vi "enum01.vi"() -> ()   [LabVIEW 2020]
panel:
  in  "Enum":T1(ring)
  in  "Numeric 2":dbl
  in  "Numeric":dbl
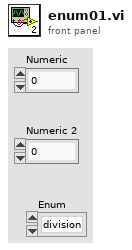
[diagram p1: front panel]
types:
  T1 = enum16{"division", "multiplicacion", "resta", "suma"}
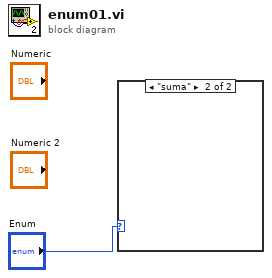
[diagram p0: block diagram]
diagram:
  n1 = case shown="\"suma\"" "Enum" {
    frame "suma", Default {
    }
    frame "suma" {
    }
  }
